vi "example_simple_qa_html_ui.vi"   [LabVIEW 2020]
uses:
  src/models/llm_openai_chatmodels/llm_openai_chatmodels.lvclass
  D:/Personal/LabVIEW LLMs/src/models/abstract_llm_base/abstract_llm_base.lvclass
  src/vectorstore/vector_qdrant/vector_qdrant.lvclass
  D:/Personal/LabVIEW LLMs/src/vectorstore/abstract_vector_base/abstract_vector_base.lvclass
  src/models/llm_openai_embedding/llm_openai_embedding.lvclass
  src/models/llm_openai_chatmodels/Instantiate_llm_openai.vi
  src/models/llm_openai_embedding/Instantiate_llm_openai_embed.vi
  src/agent/agent_simple_qa/agent_simple_qa.lvclass
  src/utilities/env_variables/env_variables.lvlib
  src/user_interfaces/simple_html_chat_ui/simple_html_chat_ui.lvclass
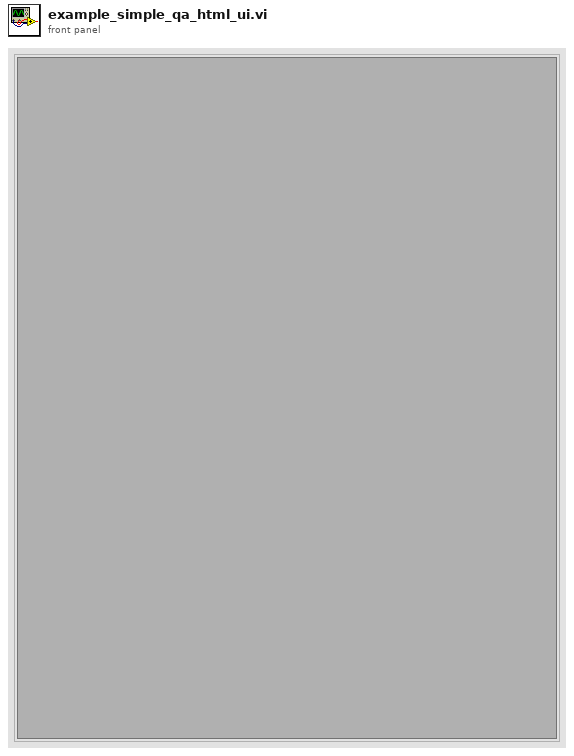
[diagram p1: front panel]
types:
  T1 = typedef "simple_html_chat_ui.lvclass/web_events.ctl" = cluster{"User prompt":refnum<user-event>, "Clear history":refnum<user-event>}
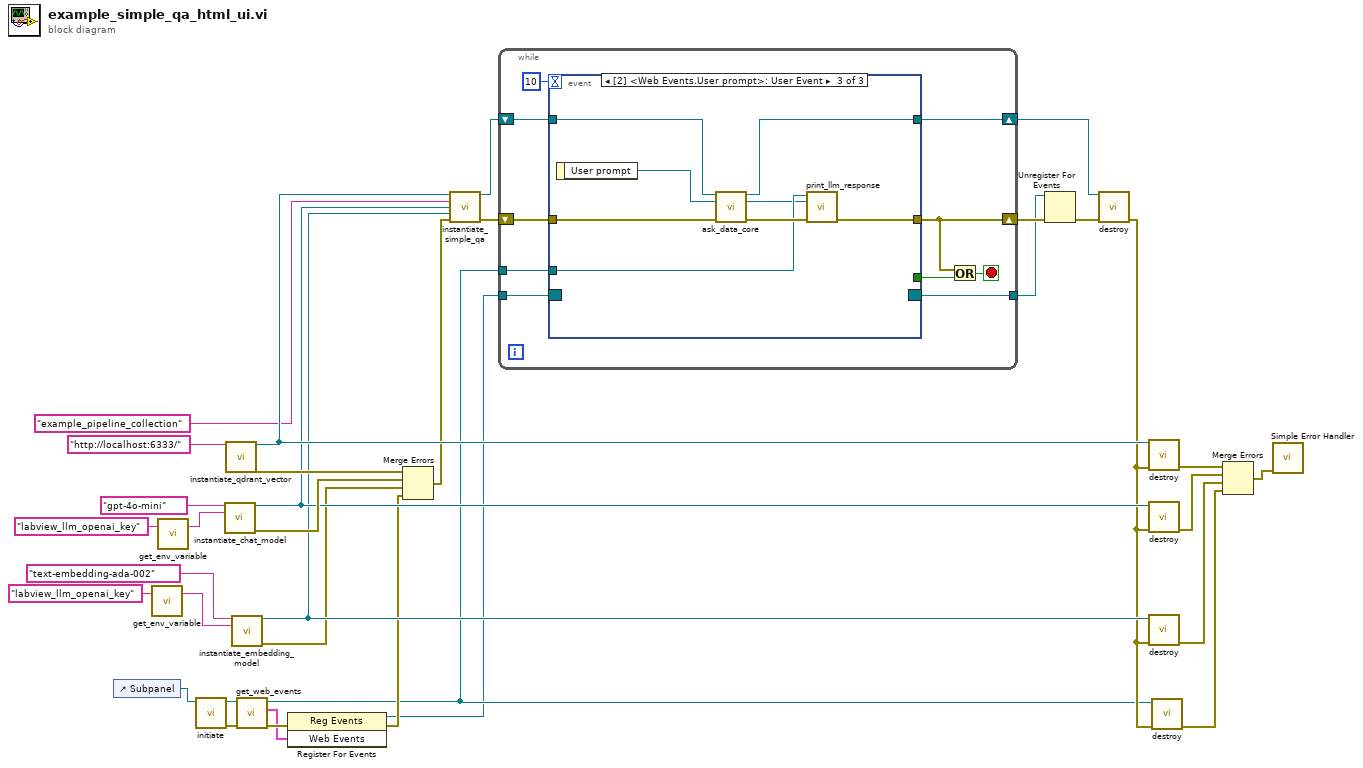
[diagram p0: block diagram]
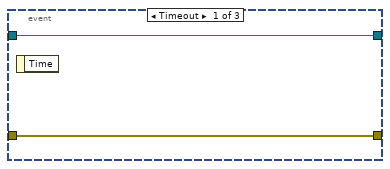
[diagram p2: hidden frame]
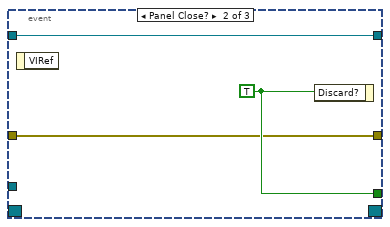
[diagram p3: hidden frame]
diagram:
  n1 = control-ref of="Subpanel"() -> (w11:refnum<vi>)
  n2 = call "get_env_variable.vi"("Environment Variable Name"="labview_llm_openai_key") -> ("Value"=w17:string)  [unwired: 1 in, 1 out]
  n3 = call "get_env_variable.vi"("Environment Variable Name"="labview_llm_openai_key") -> ("Value"=w30:string)  [unwired: 1 in, 1 out]
  n4 = call "initiate.vi"("Sub Panel"=w11) -> ("error out"=w8:errorcluster, "simple_html_chat_ui out"=w7:refnum<class "simple_html_chat_ui.lvclass">)  [unwired: 9 in]
  n5 = call-poly "instantiate_chat_model.vi"("model_name"="gpt-4o-mini", "openai_key"=w30) -> ("llm_openai out"=w21:refnum<class "llm_openai_chatmodels.lvclass">, "error out"=w23:errorcluster)  [unwired: 12 in]
  n6 = call "instantiate_qdrant_vector.vi"("host_url"="http://localhost:6333/") -> ("vector_qdrant out"=w28:refnum<class "vector_qdrant.lvclass">, "error out"=w24:errorcluster)  [unwired: 13 in]
  n7 = call-poly "instantiate_embedding_model.vi"("model_name"="text-embedding-ada-002", "openai_key"=w17) -> ("llm_openai_embedding out"=w16:refnum<class "llm_openai_embedding.lvclass">, "error out"=w15:errorcluster)  [unwired: 12 in]
  n8 = call "get_web_events.vi"("error in (no error)"=w8, "simple_html_chat_ui in"=w7) -> ("error out"=w10:errorcluster, "Web Events"=w9:T1, "simple_html_chat_ui out"=w5:refnum<class "simple_html_chat_ui.lvclass">)  [unwired: 7 in]
  n9 = register-events(error in=w10, w9) -> (reference out=w4:refnum<event-registration>, error out=w6:errorcluster)  [unwired: 1 in]
  n10 = Merge Errors(w24, w23, w15, w6) -> (w22:errorcluster)
  n11 = call "instantiate_simple_qa.vi"("vectorestore"=w28, "collection_name"="example_pipeline_collection" ("host_url"), "chat_model"=w21, "embedding_model"=w16, "error in (no error)"=w22) -> ("agent_simple_qa out"=w35:refnum<class "agent_simple_qa.lvclass">, "error out"=w34:errorcluster)  [unwired: 9 in]
  n12 = while {
    shift-right: [w42] -> w33
    shift-left: w35 -> [w43]
    shift-right: [w39] -> w3
    shift-left: w34 -> [w41]
    tunnel: w5 -> [w38]
    tunnel: w4 -> [w37]
    tunnel: [w36] -> w1
    stop <- w40 stop-if-true
    n13 = event shown="[2] <Web Events.User prompt>: User Event" {
      selector: w37 -> [_ _ _]
      dyn-events: [_ _ _] -> w36
      timeout: 10 -> [_ _ _]
      tunnel: [_ w50 _] -> w45
      tunnel: w43 -> [w46 w49 w58]
      tunnel: [w46 w49 w57] -> w42
      tunnel: w41 -> [w47 w48 w56]
      tunnel: [w47 w48 w54] -> w39
      tunnel: w38 -> [_ _ w53]
      event Timeout {
        n14 = event-data() -> ()  [unwired: 1 in, 1 out]
      }
      event Panel Close? {
        w50 = TRUE ("Discard?")
        n15 = event-data() -> ()  [unwired: 1 in, 1 out]
        n16 = event-data("Discard?"=w50) -> ()  [unwired: 1 in, 1 out]
      }
      event User Event {
        n17 = event-data() -> ("User prompt"=w51:refnum<class "abstract_message_base.lvclass">)  [unwired: 1 in]
        n18 = call-dynamic "ask_data_core.vi"("agent_simple_qa in"=w58, "message"=w51, "error in (no error)"=w56) -> ("agent_simple_qa out"=w57:refnum<class "agent_simple_qa.lvclass">, "assisstant_response"=w52:refnum<class "abstract_message_base.lvclass">, "error out"=w55:errorcluster)  [unwired: 10 in]
        n19 = call "print_llm_response.vi"("error in (no error)"=w55, "llm_response"=w52, "simple_html_chat_ui in"=w53) -> ("error out"=w54:errorcluster)  [unwired: 7 in, 1 out]
      }
    }
    n20 = Or(x=w39, y=w45) -> (x .or. y?=w40:bool)
  }
  n21 = Unregister For Events(event registration refnum=w1, error in=w3) -> (error out=w2:errorcluster)
  n22 = call-dynamic "destroy.vi"("agent_simple_qa in"=w33, "error in (no error)"=w2) -> ("error out"=w13:errorcluster)  [unwired: 12 in, 1 out]
  n23 = call-dynamic "destroy.vi"("vector_qdrant in"=w28, "error in (no error)"=w13) -> ("error out"=w27:errorcluster)  [unwired: 12 in, 1 out]
  n24 = call-dynamic "destroy.vi"("error in (no error)"=w13, "abstract_llm_base in"=w21) -> ("error out"=w26:errorcluster)  [unwired: 8 in, 1 out]
  n25 = call-dynamic "destroy.vi"("error in (no error)"=w13, "llm_openai_embedding in"=w16) -> ("error out"=w14:errorcluster)  [unwired: 8 in, 1 out]
  n26 = call "destroy.vi"("error in (no error)"=w13, "simple_html_chat_ui in"=w5) -> ("error out"=w12:errorcluster)  [unwired: 8 in, 1 out]
  n27 = Merge Errors(w27, w26, w14, w12) -> (w25:errorcluster)
  n28 = call <vilib>:"Simple Error Handler.vi"("error in (no error)"=w25) -> ()  [unwired: 4 in, 5 out]
